vi "1.0.0_Initialisation.vi"(7 "Data in":T1, 8 "error in (no error)":errorcluster, 9 "AllControls In":T2, 10 "?":T3, 11 "Message Queue out":T4) -> (0 "error out":errorcluster, 1 "Flow":string, 2 "Data":T3, 3 "Message Queue Out":T4, 5 "Data out":T1)   [LabVIEW 2017]
uses:
  Depends/AMC/subVIs/TypeDefs/amc_Message Queue.ctl
  Depends/AMC/subVIs/TypeDefs/amc_Message.ctl
  Depends/Tools/Keyed Array/Tools_KeyedArray KeyedArray.ctl
  Ctrls/Data.ctl
  Ctrls/AllControls.ctl
  Ctrls/CSV_Data.ctl
types:
  T1 = typedef "CSV_Data.ctl" = cluster{"SN":string, "Table":string[][], "Count":cluster{"Total":i32, "OK":i32, "NG":i32, "Yield":dbl}, "Start Time":timestamp, "daemon reference":refnum<k5>, "CT":dbl, "OK/NG":bool, "Station ID":string, "MES DDM SN":string, "MES PCBA SN":string, "Retest":string, "Attachment RFID detection":cluster{"UID":string, "tag content":string}, "SKU":string, "Plate_Diameter":string, "Alarm":string}
  T2 = typedef "AllControls.ctl" = cluster{"MainVI":refnum<vi>, "AlarmInfo":refnum<vi>, "Log":refnum<vi>, "Current CT":refnum<vi>, "ProductID":refnum<vi>, "Device state":refnum<vi>, "MES":refnum<vi>, "mode":refnum<vi>, "TestInfo":refnum<vi>, "SubPnl":refnum<vi>, "Table":refnum<vi>, "MES bool":refnum<vi>, "TestMode":refnum<vi>, "Recipe":refnum<vi>, "Fail resume":refnum<vi>, "LogIn":refnum<vi>, "Start":refnum<vi>, "Maintenance":refnum<vi>, "Stop":refnum<vi>, "Exit":refnum<vi>}
  T3 = typedef "Data.ctl" = cluster{"Initialisation":cluster{"DDM_Parameter":dbl[], "DDM_Parameter_status":bool[], "Get_Tester_Parameter":dbl[], "Get_Tester_Parameter_status":bool[], "Cal_Tester_Parameter":dbl[], "Cal_Tester_Parameter_status":bool[], "sw_version_before_status":bool, "sw_version_after_status":bool, "Set_SKU_Config_With_LMT_status":bool, "FCT_timestamp_status":bool, "LMT_Connect_to_UUT_status":bool}, "BEMF_Calibration":cluster{"Read_ambient_temperature":dbl, "Calibration_Vaule":dbl[], "Calibration_Vaule _B":dbl[], "Calibration_Vaule_status":bool[], "Calibration_Vaule_B_status":bool[]}, "ECO":cluster{"DDM_Parameter":dbl[], "DDM_Parameter_status":bool[], "Get_Tester_Parameter":dbl[], "Get_Tester_Parameter_status":bool[], "Cal_Tester_Parameter":dbl[], "Cal_Tester_Parameter_status":bool[], "DDM_Parameter_after_power_tune":dbl[], "Get_Tester_Parameter_after_power_tune":dbl[], "Cal_Tester_Parameter_after_power_tune":dbl[], "Cal_Tester_Parameter_after_power_tune_status":bool[], "Delta_P":dbl}, "BOOST":cluster{"DDM_Parameter":dbl[], "DDM_Parameter_status":bool[], "Get_Tester_Parameter":dbl[], "Get_Tester_Parameter_status":bool[], "Cal_Tester_Parameter":dbl[], "Cal_Tester_Parameter_status":bool[], "DDM_Parameter_after_power_tune":dbl[], "Get_Tester_Parameter_after_power_tune":dbl[], "Cal_Tester_Parameter_after_power_tune":dbl[], "Cal_Tester_Parameter_after_power_tune_status":bool[], "airwatts_am_off":dbl, "AW_Delta_(AM_on_and_off)":dbl, "AW_Delta_(AM_on_and_off)_Status":bool, "Delta_P":dbl}, "MAX":cluster{"Average_Tmag_Data":cluster{"LSI Delta in degC":dbl, "FISF Delta in degc":dbl, "LSI Tmag in degC":dbl, "Fisf Tmag in degC":dbl, "IIR Tmag in degC":dbl}, "DDM_Parameter":dbl[], "DDM_Parameter_status":bool[], "Get_Tester_Parameter":dbl[], "Get_Tester_Parameter_status":bool[], "Cal_Tester_Parameter":dbl[], "BEMF_Finetune":cluster{"eol_bemf_mp_cold_coef_c":dbl, "eol_cold_bemf_fisf_offset":dbl}, "AW_Tune":cluster{"delta_P1":dbl, "delta_P_Setting":dbl}, "DDM_Parameter_after_Airwatts_Tune":dbl[], "Get_Tester_Parameter_after_Airwatts_Tune":dbl[], "Cal_Tester_Parameter_after_Airwatts_Tune":dbl[], "DDM_Parameter_after_Airwatts_Finetune":dbl[], "Get_Tester_Parameter_after_Airwatts_Finetune":dbl[], "Cal_Tester_Parameter_after_Airwatts_Finetune":dbl[], "AW_Finetune":cluster{"delta_P2":dbl, "delta_P_Setting":dbl}, "Delta_Tmag_after_tune":cluster{"LSI Delta in degC":dbl, "FISF Delta in degc":dbl, "LSI Tmag in degC":dbl, "Fisf Tmag in degC":dbl, "IIR Tmag in degC":dbl}, "Hot Bemf in mV":dbl, "DDM_Pressure":dbl, "Delta_Pressure":dbl, " Cold Bemf in mV":dbl, " delta Bemf":dbl, " delta p":dbl, "Delta_Pressure_status":bool, " delta Bemf_status":bool, "LSI Delta in degC_status":bool, "FISF Delta in degc_status":bool, "Max_check_derate_status_status":bool, "Average_All_data":dbl[][], "Average_Tmag_Data_status":bool[], "Average_Tmag_Data_after_tune_status":bool[], "Cal_Tester_Parameter_status":bool[], "Cal_Tester_Parameter_status_after_Airwatts_Tune":bool[], "Cal_Tester_Parameter_status_after_Airwatts_FineTune":bool[]}, "Task_Detect_Calib":cluster{"LL":cluster{"DDM_Parameter":dbl[], "DDM_Parameter_status":bool[], "Get_Tester_Parameter":dbl[], "Get_Tester_Parameter_status":bool[], "Set_task_detect_A":dbl, "Set_task_detect_A_Status":bool}, "HL":cluster{"DDM_Parameter":dbl[], "DDM_Parameter_status":bool[], "Get_Tester_Parameter":dbl[], "Get_Tester_Parameter_status":bool[], "Set_task_detect_B":dbl, "Set_task_detect_B_Status":bool}, "LH":cluster{"DDM_Parameter":dbl[], "DDM_Parameter_status":bool[], "Get_Tester_Parameter":dbl[], "Get_Tester_Parameter_status":bool[], "Set_task_detect_C":dbl, "Set_task_detect_C_Status":bool}, "HH":cluster{"DDM_Parameter":dbl[], "DDM_Parameter_status":bool[], "Get_Tester_Parameter":dbl[], "Get_Tester_Parameter_status":bool[], "Set_task_detect_D":dbl, "Read_and_check_calibration_Status":bool[], "Set_task_detect_D_Status":bool}, "Get_eol_inlet_blockage_E":dbl, "Calib_vaule":cluster{"Get_task_detect_LL":dbl, "Get_task_detect_HL":dbl, "Get_task_detect_LH":dbl, "Get_task_detect_HH":dbl, "eol_inlet_blockage":dbl, "eol_code_bemf_temp":dbl}, "calibrated temp":dbl, "Inlet_Blockage_Calibration":cluster{"DDM_Parameter":dbl[], "DDM_Parameter_status":bool[], "Get_Tester_Parameter":dbl[], "Get_Tester_Parameter_status":bool[]}, "Get_eol_inlet_blockage_E_Status":bool}, "good":cluster{"Write_Product_TS":cluster{"TIMESTAMP":i64, "RIG_ID":i64, "PASSMARK_ID":i64, "PASSMARK_REV":i64}, "Read_Product_TS":cluster{"TIMESTAMP":i64, "RIG_ID":i64, "PASSMARK_ID":i64, "PASSMARK_REV":i64}, "Good_Check_Secuity_Bit_Stauts":bool}}
  T4 = typedef "amc_Message Queue.ctl" = refnum<queue>
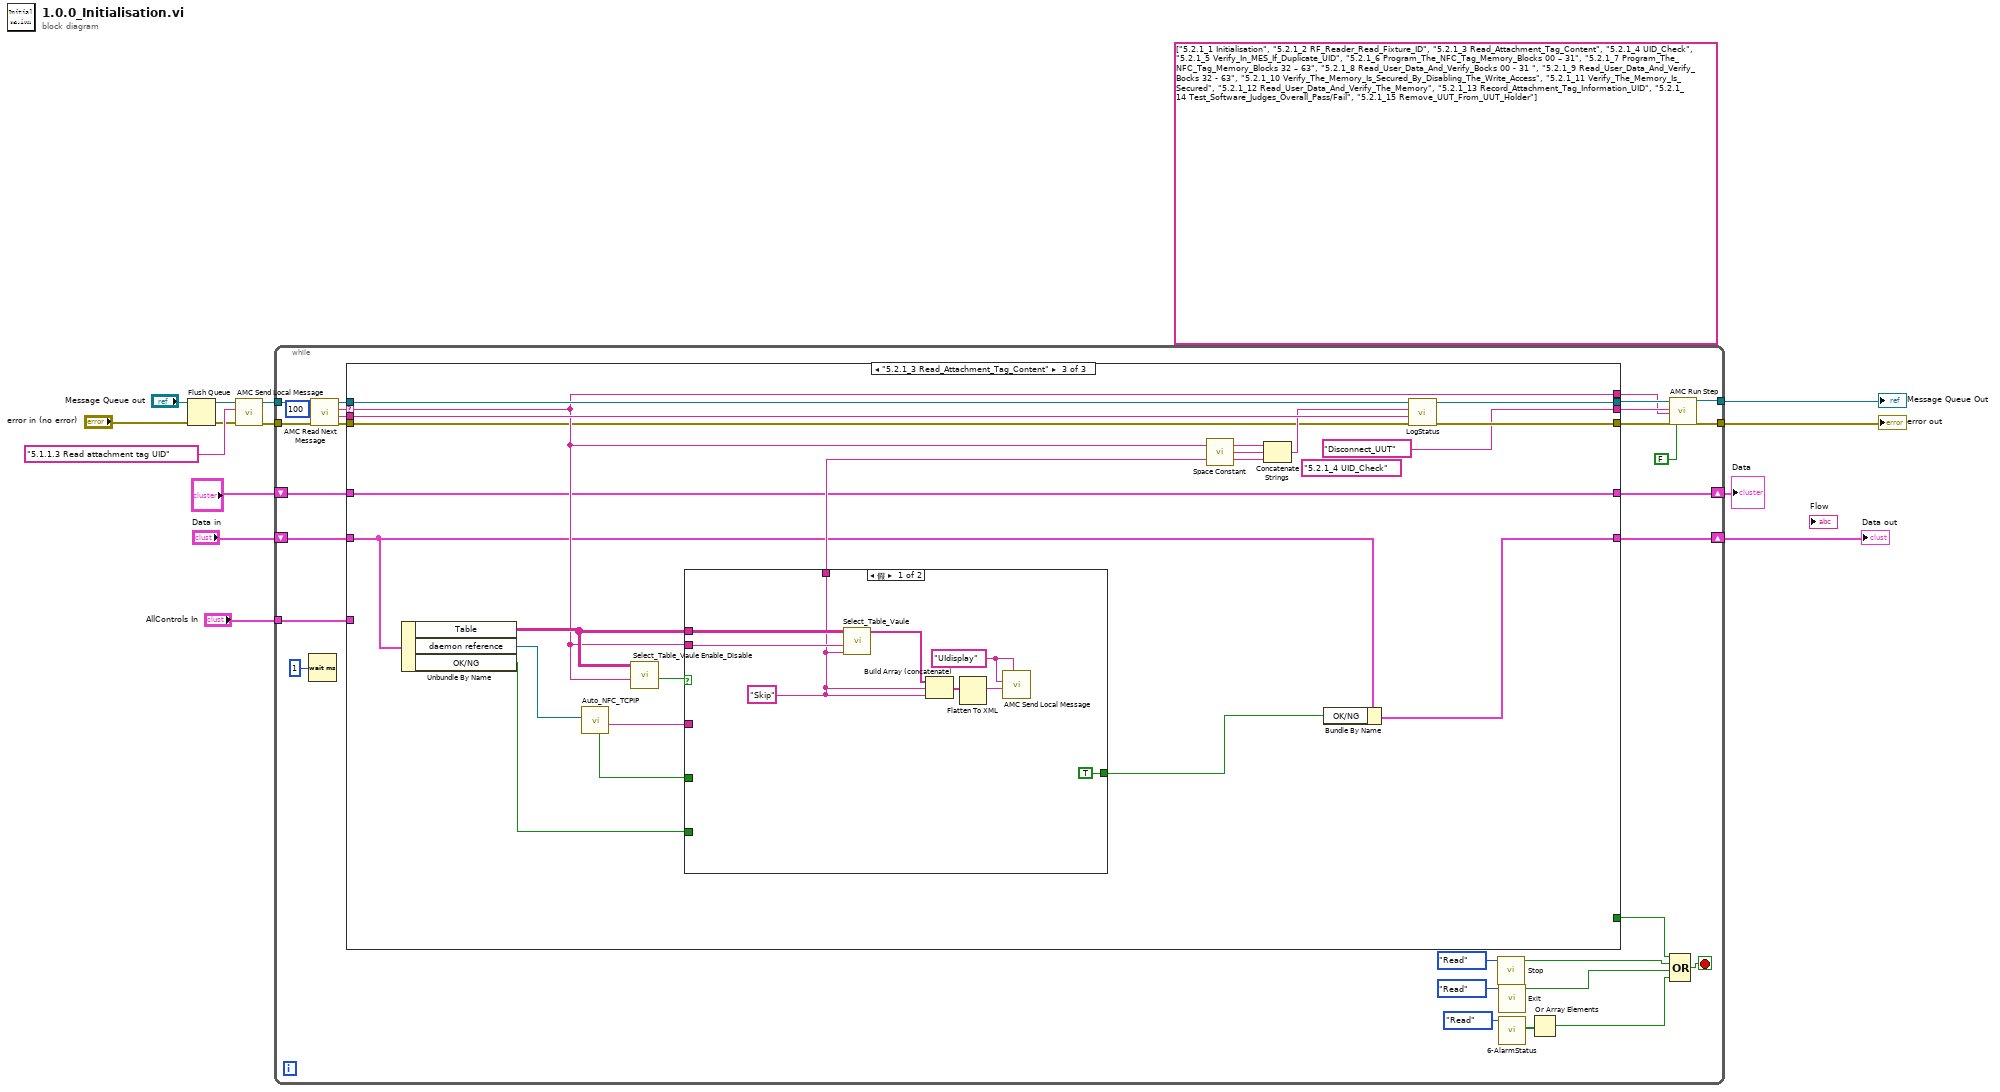
[diagram p0: block diagram]
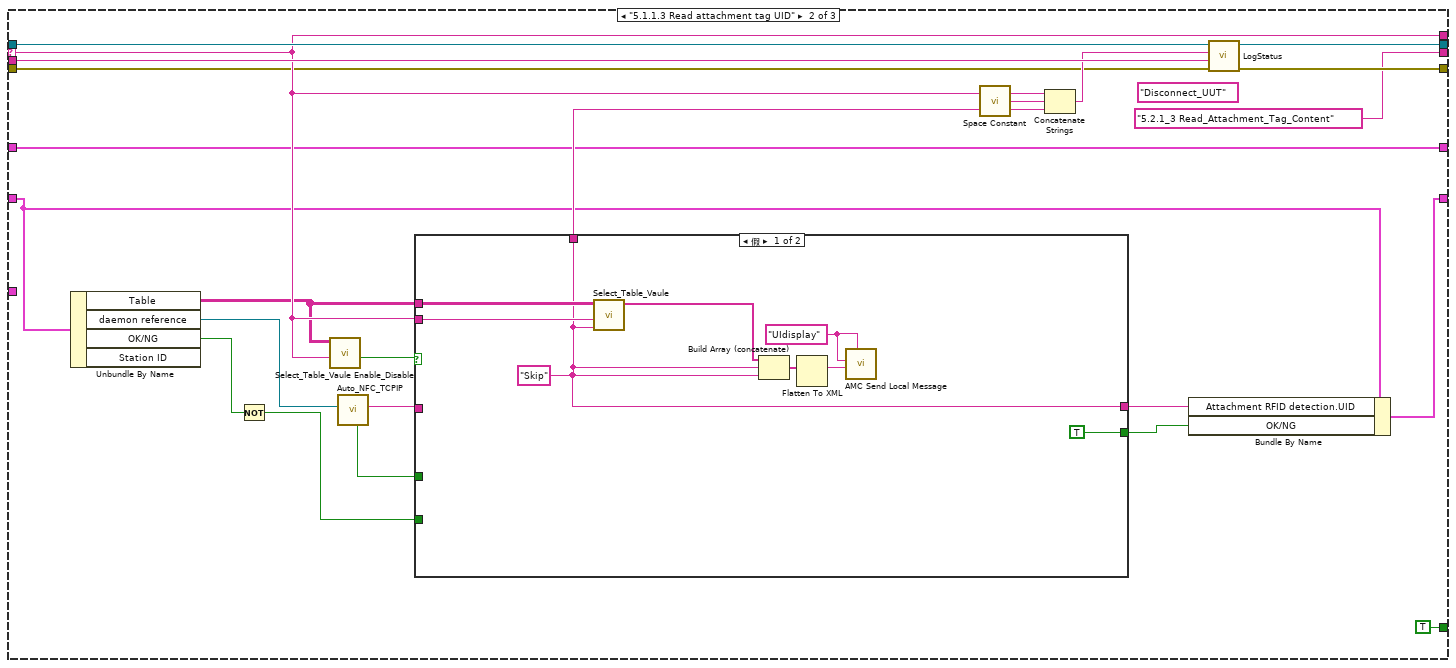
[diagram p3: hidden frame]
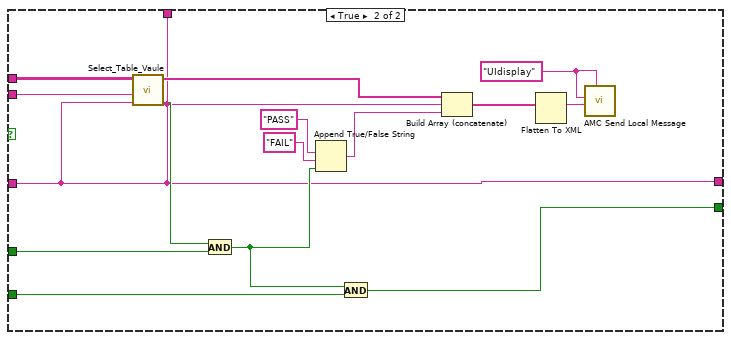
[diagram p4: hidden frame]
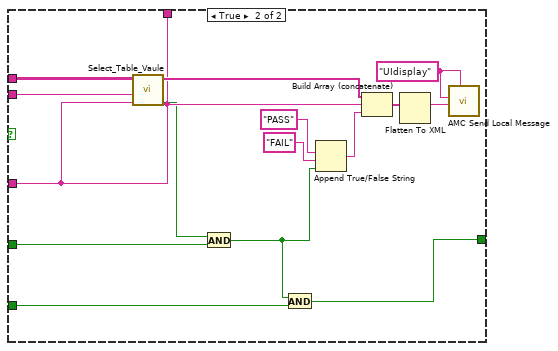
[diagram p5: hidden frame]
diagram:
  (unwired) string[] ["5.2.1_1 Initialisation", "5.2.1_2 RF_Reader_Read_Fixture_ID", "5.2.1_3 Read_Attachment_Tag_Content", "5.2.1_4 UID_Check", "5.2.1_5 Verify_In_MES_If_Duplicate_UID", "5.2.1_6 Program_The_NFC_Tag_Memory_Blocks 00 – 31", "5.2.1_7 Program_The_NFC_Tag_Memory_Blocks 32 – 63", "5.2.1_8 Read_User_Data_And_Verify_Bocks 00 - 31 ", "5.2.1_9 Read_User_Data_And_Verify_Bocks 32 - 63", "5.2.1_10 Verify_The_Memory_Is_Secured_By_Disabling_The_Write_Access", "5.2.1_11 Verify_The_Memory_Is_Secured", "5.2.1_12 Read_User_Data_And_Verify_The_Memory", "5.2.1_13 Record_Attachment_Tag_Information_UID", "5.2.1_14 Test_Software_Judges_Overall_Pass/Fail", "5.2.1_15 Remove_UUT_From_UUT_Holder"] ("subarray")
  n1 = Flush Queue(queue="Message Queue out") -> (queue out=w6:T4)  [unwired: 1 in, 2 out]
  n2 = call "AMC Send Local Message.vi"("error in (no error)"="error in (no error)", "Message Name"="5.1.1.3 Read attachment tag UID", "Message Queue in"=w6) -> ("error out"=w10:errorcluster, "Message Queue out"=w11:T4)  [unwired: 7 in]
  n3 = while {
    tunnel: w11 -> [w42]
    tunnel: [w38] -> w5
    tunnel: w10 -> [w36]
    tunnel: [w33] -> w4
    shift-right: [w29] -> w7
    shift-left: "?" -> [w30]
    tunnel: "AllControls In" -> [w19]
    shift-right: [w17] -> w1
    shift-left: "Data in" -> [w18]
    stop <- w22 stop-if-true
    n4 = Wait (ms)(milliseconds to wait=u32 1 ("等待时间（毫秒）")) -> ()  [unwired: 1 out]
    n5 = call "AMC Read Next Message.vi"("error in (no error)"=w36, "timeout (1ms)"=100, "Message Queue in"=w42) -> ("error out"=w35:errorcluster, "Message Value"=w27:string, "Message Name"=w40:string, "Message Queue out"=w41:T4)  [unwired: 1 in, 4 out]
    n6 = case shown="\"5.2.1_3 Read_Attachment_Tag_Content\"" w40 {
      selector: w40 -> [_ w63 w104]
      tunnel: w41 -> [w46 w68 w110]
      tunnel: [w46 w68 w110] -> w39
      tunnel: w35 -> [w45 w62 w103]
      tunnel: [w45 w67 w109] -> w34
      tunnel: [_ TRUE ("GRR") _] -> w23
      tunnel: w30 -> [w44 w60 w100]
      tunnel: [w44 w60 w100] -> w29
      tunnel: w27 -> [_ w66 w108]
      tunnel: [_ w63 w104] -> w26
      tunnel: [_ "5.2.1_3 Read_Attachment_Tag_Content" "Disconnect_UUT"] -> w28
      tunnel: w19 -> [_ _ _]
      tunnel: w18 -> [w43 w59 w99]
      tunnel: [w43 w58 w98] -> w17
      frame "假", Default {
      }
      frame "5.1.1.3 Read attachment tag UID" {
        (unwired) "Disconnect_UUT"
        n7 = Unbundle By Name(w59) -> ("Table"=w56:string[][], "daemon reference"=w55:refnum<k5>, "OK/NG"=w51:bool)  [unwired: 1 out]
        n8 = Not(x=w51) -> (.not. x?=w50:bool)
        n9 = call "Select_Table_Vaule Enable_Disable.vi"("Action"=w63, "Table"=w56) -> ("Enable"=w48:bool)  [unwired: 8 in, 1 out]
        n10 = call "Auto_NFC_TCPIP.vi"("connection ID in"=w55) -> ("UID"=w54:string, "x .and. y?"=w53:bool)  [unwired: 6 in, 3 out]
        n11 = case shown="假" w48 {
          tunnel: [w70 w77] -> w61
          tunnel: w56 -> [w72 w85]
          tunnel: w63 -> [w71 w84]
          tunnel: w54 -> [_ w77]
          tunnel: [w70 w77] -> w57
          tunnel: w53 -> [_ w81]
          tunnel: [TRUE w78] -> w52
          tunnel: w50 -> [_ w80]
          frame False {
            w76 = "UIdisplay" ("Process (\"\" - local)")
            w70 = "Skip" ("Action")
            n12 = call "Select_Table_Vaule.vi"("Vaule"=w70, "Action"=w71, "Table"=w72) -> ("vaule"=w73:string[])  [unwired: 7 in, 1 out]
            n13 = Build Array (concatenate)(w73, w70, w70) -> (w75:string[])
            n14 = Flatten To XML(anything=w75) -> (xml string=w74:string)
            n15 = call "AMC Send Local Message.vi"("Process (\"\" - local)"=w76, "Message Value"=w74, "Message Name"=w76) -> ()  [unwired: 7 in, 2 out]
          }
          frame True {
            w90 = "UIdisplay" ("Process (\"\" - local)")
            n16 = call "Select_Table_Vaule.vi"("Vaule"=w77, "Action"=w84, "Table"=w85) -> ("Result"=w82:bool, "vaule"=w91:string[])  [unwired: 7 in]
            n17 = And(x=w82, y=w81) -> (x .and. y?=w79:bool)
            n18 = Append True/False String(1:w79, 2:"FAIL" ("真字符串"), 3:"PASS" ("真字符串")) -> (0:w83:string)  [unwired: 1 in]
            n19 = And(x=w79, y=w80) -> (x .and. y?=w78:bool)
            n20 = Build Array (concatenate)(w91, w77, w83) -> (w89:string[])
            n21 = Flatten To XML(anything=w89) -> (xml string=w88:string)
            n22 = call "AMC Send Local Message.vi"("Process (\"\" - local)"=w90, "Message Value"=w88, "Message Name"=w90) -> ()  [unwired: 7 in, 2 out]
          }
        }
        n23 = call <vilib>:"Space Constant.vi"() -> ("String"=w64:string)
        n24 = Concatenate Strings(w63, w64, w61) -> (w65:string)
        n25 = Bundle By Name(cluster=w59, "Attachment RFID detection.UID"=w57, "OK/NG"=w52) -> (w58:T1)
        n26 = call "LogStatus.vi"("error in (no error)"=w62, "last message"=w66, "message"=w65) -> ("error  out"=w67:errorcluster)  [unwired: 8 in]
      }
      frame "5.2.1_3 Read_Attachment_Tag_Content" {
        (unwired) "5.2.1_4 UID_Check"
        n27 = Unbundle By Name(w99) -> ("Table"=w105:string[][], "daemon reference"=w97:refnum<k5>, "OK/NG"=w94:bool)
        n28 = call "Auto_NFC_TCPIP.vi"("connection ID in"=w97) -> ("Read Data"=w93:string, "x .and. y?"=w96:bool)  [unwired: 6 in, 3 out]
        n29 = call "Select_Table_Vaule Enable_Disable.vi"("Action"=w104, "Table"=w105) -> ("Enable"=w101:bool)  [unwired: 8 in, 1 out]
        n30 = case shown="假" w101 {
          tunnel: [w112 w125] -> w102
          tunnel: w105 -> [w114 w127]
          tunnel: w104 -> [w113 w126]
          tunnel: w93 -> [_ w125]
          tunnel: w96 -> [_ w123]
          tunnel: [TRUE w119] -> w95
          tunnel: w94 -> [_ w121]
          frame False {
            w118 = "UIdisplay" ("Process (\"\" - local)")
            w112 = "Skip" ("Action")
            n31 = call "Select_Table_Vaule.vi"("Vaule"=w112, "Action"=w113, "Table"=w114) -> ("vaule"=w115:string[])  [unwired: 7 in, 1 out]
            n32 = Build Array (concatenate)(w115, w112, w112) -> (w117:string[])
            n33 = Flatten To XML(anything=w117) -> (xml string=w116:string)
            n34 = call "AMC Send Local Message.vi"("Process (\"\" - local)"=w118, "Message Value"=w116, "Message Name"=w118) -> ()  [unwired: 7 in, 2 out]
          }
          frame True {
            w132 = "UIdisplay" ("Process (\"\" - local)")
            n35 = call "Select_Table_Vaule.vi"("Vaule"=w125, "Action"=w126, "Table"=w127) -> ("Result"=w122:bool, "vaule"=w133:string[])  [unwired: 7 in]
            n36 = And(x=w122, y=w123) -> (x .and. y?=w120:bool)
            n37 = And(x=w120, y=w121) -> (x .and. y?=w119:bool)
            n38 = Append True/False String(1:w120, 2:"FAIL" ("真字符串"), 3:"PASS" ("真字符串")) -> (0:w124:string)  [unwired: 1 in]
            n39 = Build Array (concatenate)(w133, w125, w124) -> (w131:string[])
            n40 = Flatten To XML(anything=w131) -> (xml string=w130:string)
            n41 = call "AMC Send Local Message.vi"("Process (\"\" - local)"=w132, "Message Value"=w130, "Message Name"=w132) -> ()  [unwired: 7 in, 2 out]
          }
        }
        n42 = call <vilib>:"Space Constant.vi"() -> ("String"=w106:string)
        n43 = Concatenate Strings(w104, w106, w102) -> (w107:string)
        n44 = Bundle By Name(cluster=w99, "OK/NG"=w95) -> (w98:T1)
        n45 = call "LogStatus.vi"("error in (no error)"=w103, "last message"=w108, "message"=w107) -> ("error  out"=w109:errorcluster)  [unwired: 8 in]
      }
    }
    n46 = call "Stop.vi"("Step"=enum16{"Initial", "Write", "Read"}."Read") -> ("Stop Out"=w21:bool)  [unwired: 9 in, 1 out]
    n47 = call "Exit.vi"("Step"=enum16{"Initial", "Write", "Read"}."Read" ("step")) -> ("Exit Out"=w20:bool)  [unwired: 9 in, 1 out]
    n48 = call "6-AlarmStatus.vi"("Step"=enum16{"Initial", "Write", "Read"}."Read") -> ("AlarmValue Out"=w15:bool[])  [unwired: 9 in, 1 out]
    n49 = Or Array Elements(Boolean array=w15) -> (logical OR=w14:bool)
    n50 = call "AMC Run Step.vi"("Message Queue In"=w39, "Message Name"=w28, "Message Value"=w26, "error in (no error)"=w34, "Mli/Sig"=FALSE) -> ("Message Queue Out"=w38:T4, "error out"=w33:errorcluster)  [unwired: 13 in]
    n51 = Compound Arithmetic op=OR(w23, w21, w20, w14) -> (w22:bool)
  }
  "Message Queue Out" <- w5
  "error out" <- w4
  "Data" <- w7
  "Data out" <- w1
